vi "tdsquery.vi"(3 "Error In (No Error)":errorcluster, 4 "String to TDS":string="BUSY?", 5 "VISA Port In":refnum<visa-resource-name>) -> (0 "Error Out":errorcluster, 1 "number":i32, 2 "VISA Port Out":refnum<visa-resource-name>)   [LabVIEW 2009]
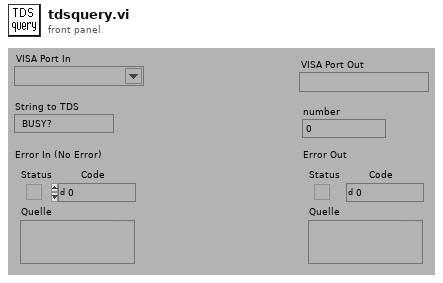
[diagram p1: front panel]
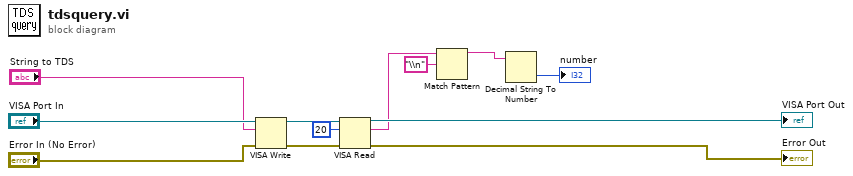
[diagram p0: block diagram]
diagram:
  n1 = VISA Write(VISA resource name="VISA Port In", write buffer="String to TDS", error in (no error)="Error In (No Error)") -> (VISA resource name out=w10:refnum<visa-resource-name>, error out=w9:errorcluster)  [unwired: 1 out]
  n2 = VISA Read(VISA resource name=w10, byte count=u32 20, error in (no error)=w9) -> (VISA resource name out=→"VISA Port Out":refnum<visa-resource-name>, read buffer=w5:string, error out=→"Error Out":errorcluster)  [unwired: 1 out]
  n3 = Match Pattern(string=w5, regular expression="\\n") -> (before substring=w3:string)  [unwired: 1 in, 3 out]
  n4 = Decimal String To Number(string=w3) -> (number=→"number":i32)  [unwired: 2 in, 1 out]
